vi "sub vi - Read Analog All v9.5.vi"(0 "data 0":waveform(dbl)[](array[waveform]), 5 "data 1":waveform(dbl)[](array[waveform]), 7 "data 2":waveform(dbl)[](array[waveform]), 9 "AI Error":errorcluster[](array[cluster])) -> (2 "Lab05 -1 Offset I":dbl, 3 "array GRAPH":dynamicdata[](array[waveform]), 4 "LAB01":T2, 6 "LAB02":T3, 8 "LAB03":T4, 10 "LAB04":T5, 13 "deg C":dbl, 14 "USB Error":bool[](array[boolean]), 15 "LAB05":T6)   [LabVIEW 2017]
uses:
  program files/Global display 3.vi
  <vilib>/measure/mascope.llb/Amplitude and Levels 1 chan.vi
  <vilib>/measure/NI_MAPro.lvlib
  <vilib>/measure/madcrms.llb/Basic Averaged DC-RMS for N Chan.vi
panel:
  in  "normalized waveform":waveform(dbl)
  in  "Tab Control":T1(tab)
  out "LAB01-2 (PF)":dbl
  out "LAB01-1 (PF)":dbl
  out "LAB01-2 (V)":dbl
  out "LAB01-2 (A)":dbl
  out "LAB01-1 (V)":dbl
  out "LAB01-1 (A)":dbl
  out "LAB01-2 (GRAPH)":dynamicdata(graph)
  out "LAB01-1 (GRAPH)":dynamicdata(graph)
  out "LAB02-2 (PF)":dbl
  out "LAB02-1 (PF)":dbl
  out "LAB02-2 (V)":dbl
  out "LAB02-2 (A)":dbl
  out "LAB02-1 (V)":dbl
  out "LAB02-1 (A)":dbl
  out "LAB02-2 (GRAPH)":dynamicdata(graph)
  out "LAB02-1 (GRAPH)":dynamicdata(graph)
  out "LAB03-2 (PF)":dbl
  out "LAB03-1 (PF)":dbl
  out "LAB03-2 (V)":dbl
  out "LAB03-2 (A)":dbl
  out "LAB03-1 (V)":dbl
  out "LAB03-1 (A)":dbl
  out "LAB03-2 (GRAPH)":dynamicdata(graph)
  out "LAB03-1 (GRAPH)":dynamicdata(graph)
  out "LAB04-2 (PF)":dbl
  out "LAB04-1 (PF)":dbl
  out "LAB04-2 (V)":dbl
  out "LAB04-2 (A)":dbl
  out "LAB04-1 (V)":dbl
  out "LAB04-1 (A)":dbl
  out "LAB04-1 (GRAPH)":dynamicdata(graph)
  out "LAB04-2 (GRAPH)":dynamicdata(graph)
  out "LAB05-2 (PF)":dbl
  out "LAB05-1 (PF)":dbl
  out "LAB05-2 (V)":dbl
  out "LAB05-2 (A)":dbl
  out "LAB05-1 (V)":dbl
  out "LAB05-1 (A)":dbl
  out "LAB05-1 (GRAPH)":dynamicdata(graph)
  out "LAB05-2 (GRAPH)":dynamicdata(graph)
  out "A1 error":errorcluster
  out "array ERROR":errorcluster[](array[cluster])
  out "AI2-OFF":waveform(dbl)[](graph)
  out "AI2-ON":waveform(dbl)[](graph)
  out "AI1-OFF":waveform(dbl)[](graph)
  out "AI1-ON":waveform(dbl)[](graph)
  out "AI0-OFF":waveform(dbl)[](graph)
  out "AI0-ON":waveform(dbl)[](graph)
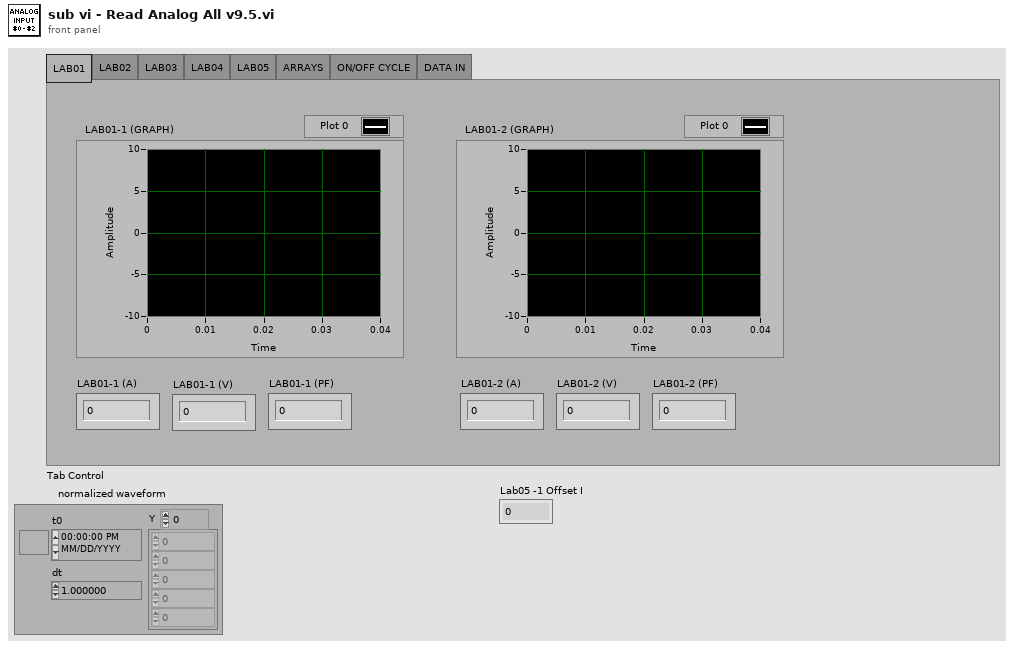
[diagram p1: front panel]
types:
  T1 = enum32{"LAB01", "LAB02", "LAB03", "LAB04", "LAB05", "ARRAYS", "ON/OFF CYCLE", "DATA IN"}
  T2 = cluster{"LAB01-1 (A)":dbl, "LAB01-1 (V)":dbl, "LAB01-1 (PF)":dbl, "LAB01-2 (A)":dbl, "LAB01-2 (V)":dbl, "LAB01-2 (PF)":dbl}
  T3 = cluster{"LAB02-1 (A)":dbl, "LAB02-1 (V)":dbl, "LAB02-1 (PF)":dbl, "LAB02-2 (A)":dbl, "LAB02-2 (V)":dbl, "LAB02-2 (PF)":dbl}
  T4 = cluster{"LAB03-1 (A)":dbl, "LAB03-1 (V)":dbl, "LAB03-1 (PF)":dbl, "LAB03-2 (A)":dbl, "LAB03-2 (V)":dbl, "LAB03-2 (PF)":dbl}
  T5 = cluster{"LAB04-1 (A)":dbl, "LAB04-1 (V)":dbl, "LAB04-1 (PF)":dbl, "LAB04-2 (A)":dbl, "LAB04-2 (V)":dbl, "LAB04-2 (PF)":dbl}
  T6 = cluster{"LAB05-1 (A)":dbl, "LAB05-1 (V)":dbl, "LAB05-1 (PF)":dbl, "LAB05-2 (A)":dbl, "LAB05-2 (V)":dbl, "LAB05-2 (PF)":dbl}
  T7 = cluster{"active power [W]":dbl, "apparent power [VA]":dbl, "reactive power [VAR]":dbl, "power factor":dbl}
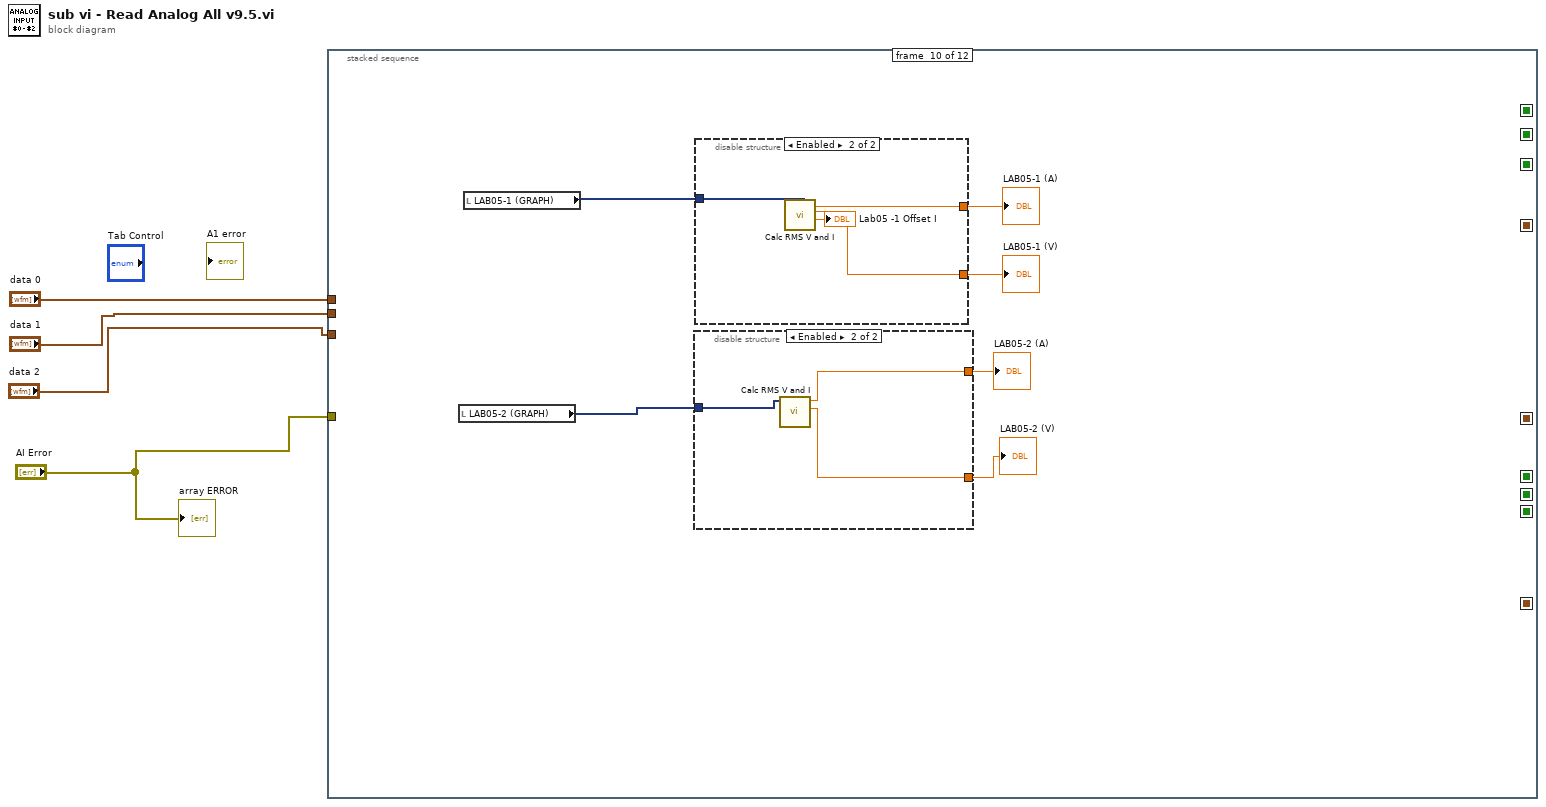
[diagram p0: block diagram]
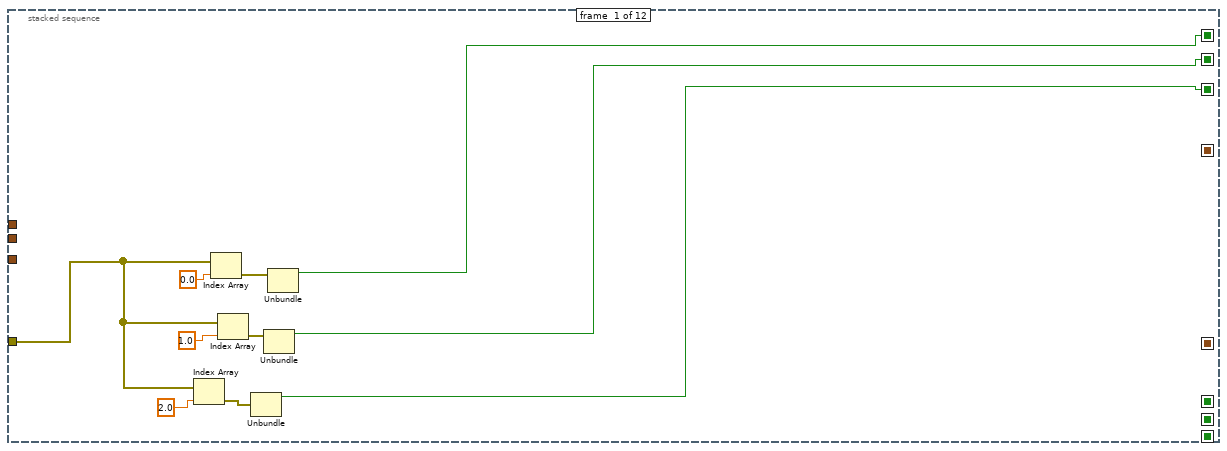
[diagram p2: hidden frame]
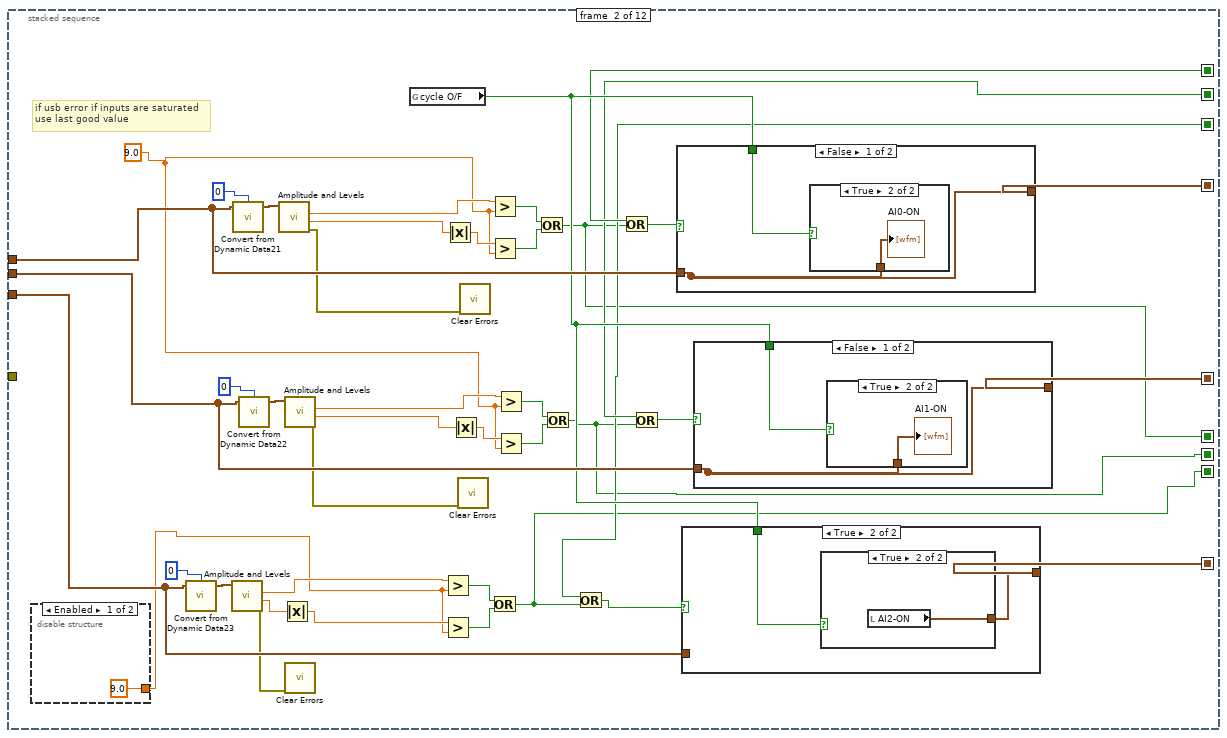
[diagram p3: hidden frame]
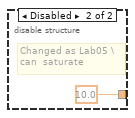
[diagram p4: hidden frame]
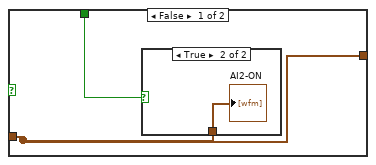
[diagram p5: hidden frame]
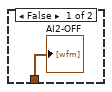
[diagram p6: hidden frame]
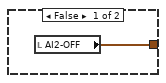
[diagram p7: hidden frame]
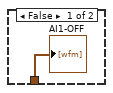
[diagram p8: hidden frame]
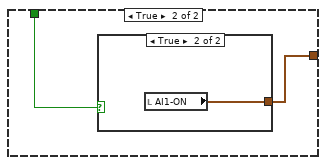
[diagram p9: hidden frame]
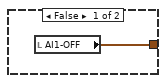
[diagram p10: hidden frame]
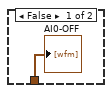
[diagram p11: hidden frame]
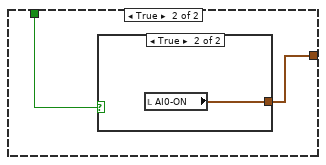
[diagram p12: hidden frame]
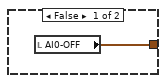
[diagram p13: hidden frame]
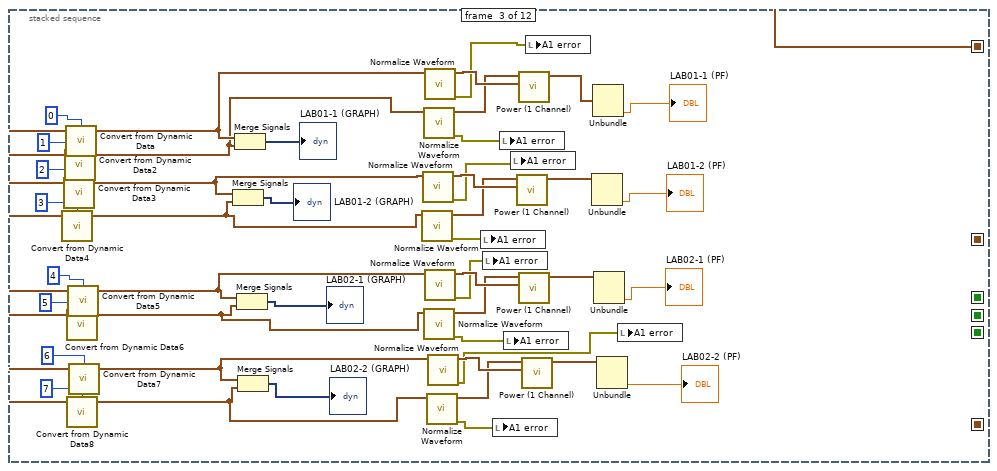
[diagram p14: hidden frame]
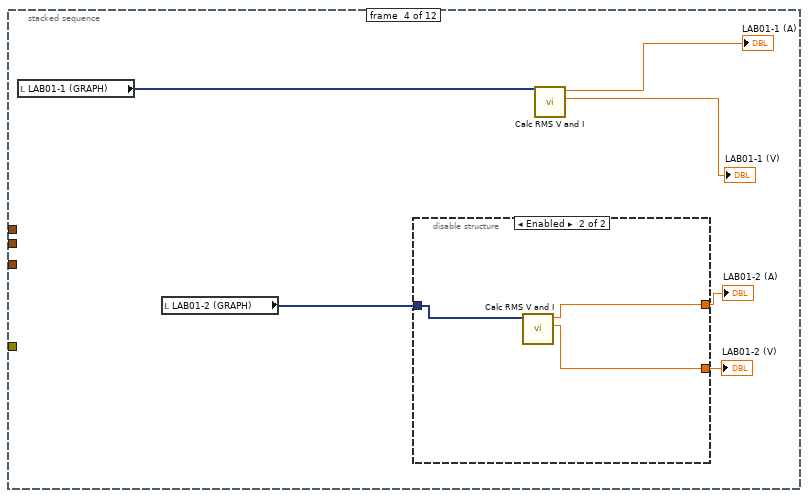
[diagram p15: hidden frame]
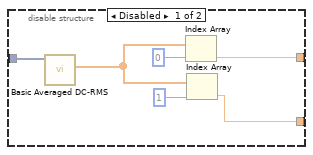
[diagram p16: hidden frame]
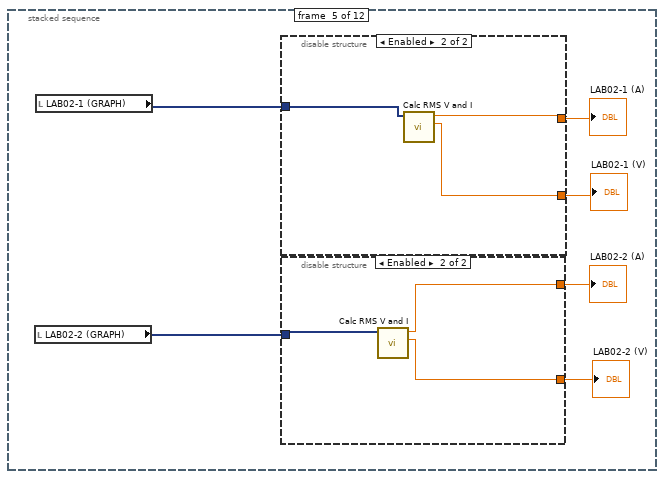
[diagram p17: hidden frame]
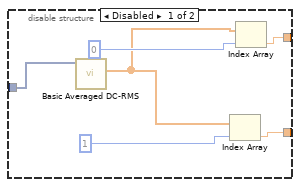
[diagram p18: hidden frame]
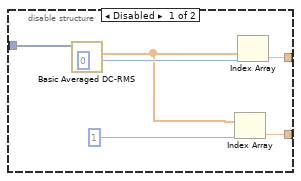
[diagram p19: hidden frame]
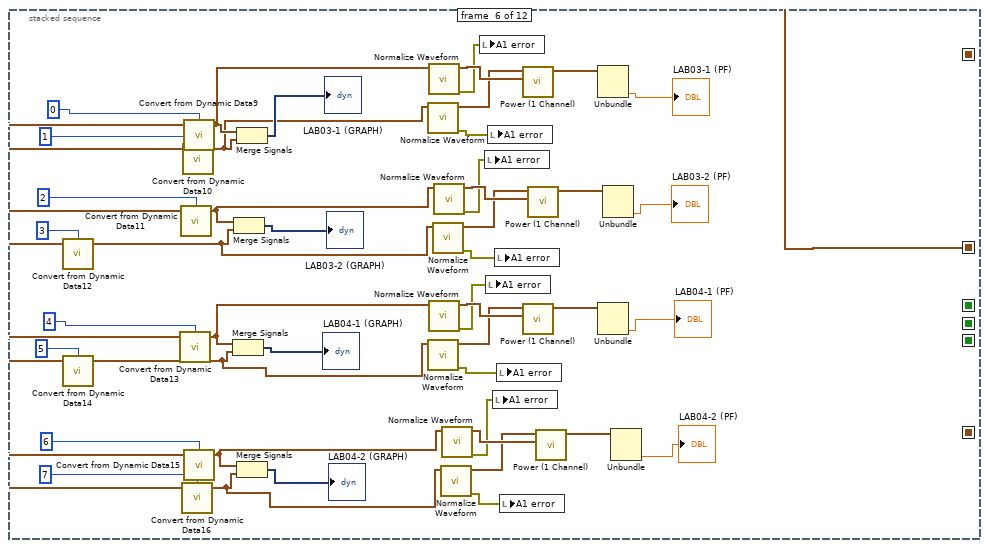
[diagram p20: hidden frame]
diagram:
  n1 = stacked-sequence {
    seq-local: [w12 _ _ _ _ _ _ _ _ _ _ _] -> [_ w24 _ _ _ _ _ _ _ _ _ w327]
    seq-local: [w9 _ _ _ _ _ _ _ _ _ _ _] -> [_ w23 _ _ _ _ _ _ _ _ _ w326]
    seq-local: [w5 _ _ _ _ _ _ _ _ _ _ _] -> [_ w20 _ _ _ _ _ _ _ _ _ w325]
    seq-local: [_ w49 _ _ _ _ _ _ _ _ _ _] -> [_ _ w127 _ _ _ _ _ _ _ _ _]
    seq-local: [_ w39 _ _ _ _ _ _ _ _ _ _] -> [_ _ _ _ _ w211 _ _ _ _ _ _]
    seq-local: [_ w29 _ _ _ _ _ _ _ _ _ _] -> [_ _ _ _ _ _ _ _ w262 _ _ _]
    seq-local: [_ w19 _ _ _ _ _ _ _ _ _ _] -> [_ _ _ _ _ _ _ _ _ _ _ w324]
    seq-local: [_ w18 _ _ _ _ _ _ _ _ _ _] -> [_ _ _ _ _ _ _ _ _ _ _ w323]
    seq-local: [_ w17 _ _ _ _ _ _ _ _ _ _] -> [_ _ _ _ _ _ _ _ _ _ _ w322]
    tunnel: "data 0" -> [_ w48 _ _ _ _ _ _ _ _ _ _]
    tunnel: "data 1" -> [_ w40 _ _ _ _ _ _ _ _ _ _]
    tunnel: "data 2" -> [_ w31 _ _ _ _ _ _ _ _ _ _]
    tunnel: "AI Error" -> [w6 _ _ _ _ _ _ _ _ _ _ _]
    frame #0 {
      n2 = Index Array(array=w6, index=2.0) -> (element=w7:errorcluster)
      n3 = Index Array(array=w6, index=0.0) -> (element=w13:errorcluster)
      n4 = Index Array(array=w6, index=1.0) -> (element=w10:errorcluster)
      n5 = Unbundle(w7) -> ("status"=w5:bool)  [unwired: 2 out]
      n6 = Unbundle(w10) -> ("status"=w9:bool)  [unwired: 2 out]
      n7 = Unbundle(w13) -> ("status"=w12:bool)  [unwired: 2 out]
    }
    frame #1 {
      w15 = 9.0
      # "if usb error if inputs are saturated\nuse last good value"
      n8 = disable-structure shown="Enabled" {
        disable-tunnel: [9.0 10.0] -> w16
        frame Enabled {
        }
        frame Disabled {
          # "Changed as Lab05 \\\ncan  saturate"
        }
      }
      n9 = call "Convert from Dynamic Data23"("Dynamic Data Type"=w31, "Channel"=0) -> ("Waveform"=w37:waveform(dbl))  [unwired: 2 in]
      n10 = call-poly <vilib>:"Amplitude and Levels.vi"("signal in"=w37) -> ("error out"=w26:errorcluster, "low state level"=w36:dbl, "high state level"=w35:dbl)  [unwired: 7 in, 1 out]
      n11 = call "Convert from Dynamic Data21"("Dynamic Data Type"=w48, "Channel"=0) -> ("Waveform"=w55:waveform(dbl))  [unwired: 2 in]
      n12 = call "Convert from Dynamic Data22"("Dynamic Data Type"=w40, "Channel"=0) -> ("Waveform"=w46:waveform(dbl))  [unwired: 2 in]
      n13 = call-poly <vilib>:"Amplitude and Levels.vi"("signal in"=w55) -> ("error out"=w28:errorcluster, "low state level"=w54:dbl, "high state level"=w53:dbl)  [unwired: 7 in, 1 out]
      n14 = Absolute Value(x=w36) -> (abs(x)=w34:dbl)
      n15 = call-poly <vilib>:"Amplitude and Levels.vi"("signal in"=w46) -> ("error out"=w27:errorcluster, "low state level"=w45:dbl, "high state level"=w44:dbl)  [unwired: 7 in, 1 out]
      n16 = call <vilib>:"Clear Errors.vi"("error in (no error)"=w26) -> ()  [unwired: 5 in, 2 out]
      n17 = global read "Global display 3.vi" "cycle O/F"() -> (w30:bool)
      n18 = Greater?(x=w35, y=w16) -> (0:w33:bool)
      n19 = Greater?(x=w34, y=w16) -> (0:w32:bool)
      n20 = Absolute Value(x=w54) -> (abs(x)=w52:dbl)
      n21 = Absolute Value(x=w45) -> (abs(x)=w43:dbl)
      n22 = call <vilib>:"Clear Errors.vi"("error in (no error)"=w27) -> ()  [unwired: 5 in, 2 out]
      n23 = call <vilib>:"Clear Errors.vi"("error in (no error)"=w28) -> ()  [unwired: 5 in, 2 out]
      n24 = Greater?(x=w53, y=w15) -> (0:w51:bool)
      n25 = Greater?(x=w52, y=w15) -> (0:w50:bool)
      n26 = Or(x=w33, y=w32) -> (x .or. y?=w17:bool)
      n27 = Greater?(x=w44, y=w15) -> (0:w42:bool)
      n28 = Greater?(x=w43, y=w15) -> (0:w41:bool)
      n29 = Or(x=w51, y=w50) -> (x .or. y?=w19:bool)
      n30 = Or(x=w42, y=w41) -> (x .or. y?=w18:bool)
      n31 = Or(x=w20, y=w17) -> (x .or. y?=w21:bool)
      n32 = Or(x=w24, y=w19) -> (x .or. y?=w25:bool)
      n33 = Or(x=w23, y=w18) -> (x .or. y?=w22:bool)
      n34 = case shown="False" w25 {
        tunnel: w30 -> [w76 w80]
        tunnel: [w75 w79] -> w49
        tunnel: w48 -> [w75 _]
        frame False {
          n35 = case shown="True" w76 {
            tunnel: w75 -> [w77 w78]
            frame False {
              "AI0-OFF" <- w77
            }
            frame True {
              "AI0-ON" <- w78
            }
          }
        }
        frame True {
          n36 = case shown="True" w80 {
            tunnel: [w81 w82] -> w79
            frame False {
              n37 = local read "AI0-OFF"() -> (w81:waveform(dbl)[])
            }
            frame True {
              n38 = local read "AI0-ON"() -> (w82:waveform(dbl)[])
            }
          }
        }
      }
      n39 = case shown="True" w21 {
        tunnel: w30 -> [w60 w64]
        tunnel: [w59 w63] -> w29
        tunnel: w31 -> [w59 _]
        frame False {
          n40 = case shown="True" w60 {
            tunnel: w59 -> [w61 w62]
            frame False {
              "AI2-OFF" <- w61
            }
            frame True {
              "AI2-ON" <- w62
            }
          }
        }
        frame True {
          n41 = case shown="True" w64 {
            tunnel: [w65 w66] -> w63
            frame False {
              n42 = local read "AI2-OFF"() -> (w65:waveform(dbl)[])
            }
            frame True {
              n43 = local read "AI2-ON"() -> (w66:waveform(dbl)[])
            }
          }
        }
      }
      n44 = case shown="False" w22 {
        tunnel: w30 -> [w68 w72]
        tunnel: [w67 w71] -> w39
        tunnel: w40 -> [w67 _]
        frame False {
          n45 = case shown="True" w68 {
            tunnel: w67 -> [w69 w70]
            frame False {
              "AI1-OFF" <- w69
            }
            frame True {
              "AI1-ON" <- w70
            }
          }
        }
        frame True {
          n46 = case shown="True" w72 {
            tunnel: [w73 w74] -> w71
            frame False {
              n47 = local read "AI1-OFF"() -> (w73:waveform(dbl)[])
            }
            frame True {
              n48 = local read "AI1-ON"() -> (w74:waveform(dbl)[])
            }
          }
        }
      }
    }
    frame #2 {
      n49 = call "Convert from Dynamic Data4"("Dynamic Data Type"=w127, "Channel"=3) -> ("Waveform"=w103:waveform(dbl))  [unwired: 2 in]
      n50 = call "Convert from Dynamic Data3"("Dynamic Data Type"=w127, "Channel"=2) -> ("Waveform"=w104:waveform(dbl))  [unwired: 2 in]
      n51 = call "Convert from Dynamic Data2"("Dynamic Data Type"=w127, "Channel"=1) -> ("Waveform"=w113:waveform(dbl))  [unwired: 2 in]
      n52 = call "Convert from Dynamic Data"("Dynamic Data Type"=w127, "Channel"=0) -> ("Waveform"=w114:waveform(dbl))  [unwired: 2 in]
      n53 = call "Convert from Dynamic Data6"("Dynamic Data Type"=w127, "Channel"=5) -> ("Waveform"=w98:waveform(dbl))  [unwired: 2 in]
      n54 = call "Convert from Dynamic Data8"("Dynamic Data Type"=w127, "Channel"=7) -> ("Waveform"=w92:waveform(dbl))  [unwired: 2 in]
      n55 = call "Convert from Dynamic Data5"("Dynamic Data Type"=w127, "Channel"=4) -> ("Waveform"=w99:waveform(dbl))  [unwired: 2 in]
      n56 = call "Convert from Dynamic Data7"("Dynamic Data Type"=w127, "Channel"=6) -> ("Waveform"=w93:waveform(dbl))  [unwired: 2 in]
      n57 = Merge Signals(w104, w103) -> (→"LAB01-2 (GRAPH)":dynamicdata)
      n58 = Merge Signals(w114, w113) -> (→"LAB01-1 (GRAPH)":dynamicdata)
      n59 = Merge Signals(w99, w98) -> (→"LAB02-1 (GRAPH)":dynamicdata)
      n60 = Merge Signals(w93, w92) -> (→"LAB02-2 (GRAPH)":dynamicdata)
      n61 = call <vilib>:"Normalize Waveform.vi"("waveform in"=w103) -> ("error out"=w87:errorcluster, "normalized waveform"=w107:waveform(dbl))  [unwired: 7 in, 2 out]
      n62 = call <vilib>:"Normalize Waveform.vi"("waveform in"=w104) -> ("error out"=w88:errorcluster, "normalized waveform"=w108:waveform(dbl))  [unwired: 7 in, 2 out]
      n63 = call <vilib>:"Normalize Waveform.vi"("waveform in"=w113) -> ("error out"=w89:errorcluster, "normalized waveform"=w111:waveform(dbl))  [unwired: 7 in, 2 out]
      n64 = call <vilib>:"Normalize Waveform.vi"("waveform in"=w98) -> ("error out"=w85:errorcluster, "normalized waveform"=w101:waveform(dbl))  [unwired: 7 in, 2 out]
      n65 = call <vilib>:"Normalize Waveform.vi"("waveform in"=w114) -> ("error out"=w90:errorcluster, "normalized waveform"=w112:waveform(dbl))  [unwired: 7 in, 2 out]
      n66 = call <vilib>:"Normalize Waveform.vi"("waveform in"=w99) -> ("error out"=w86:errorcluster, "normalized waveform"=w102:waveform(dbl))  [unwired: 7 in, 2 out]
      n67 = call <vilib>:"Normalize Waveform.vi"("waveform in"=w92) -> ("error out"=w83:errorcluster, "normalized waveform"=w95:waveform(dbl))  [unwired: 7 in, 2 out]
      n68 = call <vilib>:"Normalize Waveform.vi"("waveform in"=w93) -> ("error out"=w84:errorcluster, "normalized waveform"=w96:waveform(dbl))  [unwired: 7 in, 2 out]
      n69 = local write "A1 error"(w87) -> ()
      n70 = local write "A1 error"(w86) -> ()
      n71 = local write "A1 error"(w83) -> ()
      n72 = local write "A1 error"(w89) -> ()
      n73 = local write "A1 error"(w85) -> ()
      n74 = local write "A1 error"(w88) -> ()
      n75 = call "Power (1 Channel).vi"("current waveform"=w108, "voltage waveform"=w107) -> ("power value"=w106:T7)  [unwired: 9 in]
      n76 = call "Power (1 Channel).vi"("current waveform"=w112, "voltage waveform"=w111) -> ("power value"=w110:T7)  [unwired: 9 in]
      n77 = call "Power (1 Channel).vi"("current waveform"=w102, "voltage waveform"=w101) -> ("power value"=w100:T7)  [unwired: 9 in]
      n78 = call "Power (1 Channel).vi"("current waveform"=w96, "voltage waveform"=w95) -> ("power value"=w94:T7)  [unwired: 9 in]
      n79 = local write "A1 error"(w90) -> ()
      n80 = Unbundle(w106) -> ("power factor"=→"LAB01-2 (PF)":dbl)  [unwired: 3 out]
      n81 = Unbundle(w110) -> ("power factor"=→"LAB01-1 (PF)":dbl)  [unwired: 3 out]
      n82 = Unbundle(w100) -> ("power factor"=→"LAB02-1 (PF)":dbl)  [unwired: 3 out]
      n83 = Unbundle(w94) -> ("power factor"=→"LAB02-2 (PF)":dbl)  [unwired: 3 out]
      n84 = local write "A1 error"(w84) -> ()
    }
    frame #3 {
      n85 = local read "LAB01-1 (GRAPH)"() -> (w128:dynamicdata)
      n86 = local read "LAB01-2 (GRAPH)"() -> (w129:dynamicdata)
      n87 = disable-structure shown="Enabled" {
        disable-tunnel: [w136 w141] -> w133
        disable-tunnel: [w135 w140] -> w132
        disable-tunnel: w129 -> [w134 w142]
        frame Disabled {
          n88 = call-poly <vilib>:"Basic Averaged DC-RMS.vi"("signals in"=w134) -> ("RMS values"=w139:dbl[])  [unwired: 7 in, 3 out]
          n89 = Index Array(array=w139, index=0) -> (element=w136:dbl)
          n90 = Index Array(array=w139, index=1) -> (element=w135:dbl)
        }
        frame Enabled {
          n91 = call "Calc RMS V and I.vi"("LAB01-1 (GRAPH)"=w142) -> ("RMS V"=w140:dbl, "RMS I"=w141:dbl)  [unwired: 8 in, 1 out]
        }
      }
      "LAB01-2 (A)" <- w133
      "LAB01-2 (V)" <- w132
      n92 = call "Calc RMS V and I.vi"("LAB01-1 (GRAPH)"=w128) -> ("RMS V"=→"LAB01-1 (V)":dbl, "RMS I"=→"LAB01-1 (A)":dbl)  [unwired: 8 in, 1 out]
    }
    frame #4 {
      n93 = local read "LAB02-2 (GRAPH)"() -> (w144:dynamicdata)
      n94 = local read "LAB02-1 (GRAPH)"() -> (w143:dynamicdata)
      n95 = disable-structure shown="Enabled" {
        disable-tunnel: [w160 w165] -> w148
        disable-tunnel: [w159 w164] -> w147
        disable-tunnel: w143 -> [w158 w166]
        frame Disabled {
          n96 = call-poly <vilib>:"Basic Averaged DC-RMS.vi"("signals in"=w158) -> ("RMS values"=w161:dbl[])  [unwired: 7 in, 3 out]
          n97 = Index Array(array=w161, index=1) -> (element=w159:dbl)
          n98 = Index Array(array=w161, index=0) -> (element=w160:dbl)
        }
        frame Enabled {
          n99 = call "Calc RMS V and I.vi"("LAB01-1 (GRAPH)"=w166) -> ("RMS V"=w164:dbl, "RMS I"=w165:dbl)  [unwired: 8 in, 1 out]
        }
      }
      "LAB02-1 (A)" <- w148
      "LAB02-1 (V)" <- w147
      n100 = disable-structure shown="Enabled" {
        disable-tunnel: [w151 w156] -> w146
        disable-tunnel: [w150 w155] -> w145
        disable-tunnel: w144 -> [w149 w157]
        frame Disabled {
          n101 = call-poly <vilib>:"Basic Averaged DC-RMS.vi"("signals in"=w149) -> ("RMS values"=w152:dbl[])  [unwired: 7 in, 3 out]
          n102 = Index Array(array=w152, index=1) -> (element=w150:dbl)
          n103 = Index Array(array=w152, index=0) -> (element=w151:dbl)
        }
        frame Enabled {
          n104 = call "Calc RMS V and I.vi"("LAB01-1 (GRAPH)"=w157) -> ("RMS V"=w155:dbl, "RMS I"=w156:dbl)  [unwired: 8 in, 1 out]
        }
      }
      "LAB02-2 (A)" <- w146
      "LAB02-2 (V)" <- w145
    }
    frame #5 {
      n105 = call "Convert from Dynamic Data12"("Dynamic Data Type"=w211, "Channel"=3) -> ("Waveform"=w188:waveform(dbl))  [unwired: 2 in]
      n106 = call "Convert from Dynamic Data14"("Dynamic Data Type"=w211, "Channel"=5) -> ("Waveform"=w182:waveform(dbl))  [unwired: 2 in]
      n107 = call "Convert from Dynamic Data13"("Dynamic Data Type"=w211, "Channel"=4) -> ("Waveform"=w183:waveform(dbl))  [unwired: 2 in]
      n108 = call "Convert from Dynamic Data11"("Dynamic Data Type"=w211, "Channel"=2) -> ("Waveform"=w189:waveform(dbl))  [unwired: 2 in]
      n109 = call "Convert from Dynamic Data16"("Dynamic Data Type"=w211, "Channel"=7) -> ("Waveform"=w176:waveform(dbl))  [unwired: 2 in]
      n110 = call "Convert from Dynamic Data10"("Dynamic Data Type"=w211, "Channel"=1) -> ("Waveform"=w194:waveform(dbl))  [unwired: 2 in]
      n111 = call "Convert from Dynamic Data9"("Dynamic Data Type"=w211, "Channel"=0) -> ("Waveform"=w195:waveform(dbl))  [unwired: 2 in]
      n112 = call "Convert from Dynamic Data15"("Dynamic Data Type"=w211, "Channel"=6) -> ("Waveform"=w177:waveform(dbl))  [unwired: 2 in]
      n113 = Merge Signals(w183, w182) -> (→"LAB04-1 (GRAPH)":dynamicdata)
      n114 = Merge Signals(w189, w188) -> (→"LAB03-2 (GRAPH)":dynamicdata)
      n115 = Merge Signals(w195, w194) -> (→"LAB03-1 (GRAPH)":dynamicdata)
      n116 = Merge Signals(w177, w176) -> (→"LAB04-2 (GRAPH)":dynamicdata)
      n117 = call <vilib>:"Normalize Waveform.vi"("waveform in"=w194) -> ("error out"=w173:errorcluster, "normalized waveform"=w197:waveform(dbl))  [unwired: 7 in, 2 out]
      n118 = call <vilib>:"Normalize Waveform.vi"("waveform in"=w182) -> ("error out"=w169:errorcluster, "normalized waveform"=w185:waveform(dbl))  [unwired: 7 in, 2 out]
      n119 = call <vilib>:"Normalize Waveform.vi"("waveform in"=w195) -> ("error out"=w174:errorcluster, "normalized waveform"=w198:waveform(dbl))  [unwired: 7 in, 2 out]
      n120 = call <vilib>:"Normalize Waveform.vi"("waveform in"=w183) -> ("error out"=w170:errorcluster, "normalized waveform"=w186:waveform(dbl))  [unwired: 7 in, 2 out]
      n121 = call <vilib>:"Normalize Waveform.vi"("waveform in"=w188) -> ("error out"=w171:errorcluster, "normalized waveform"=w191:waveform(dbl))  [unwired: 7 in, 2 out]
      n122 = call <vilib>:"Normalize Waveform.vi"("waveform in"=w189) -> ("error out"=w172:errorcluster, "normalized waveform"=w192:waveform(dbl))  [unwired: 7 in, 2 out]
      n123 = call <vilib>:"Normalize Waveform.vi"("waveform in"=w176) -> ("error out"=w167:errorcluster, "normalized waveform"=w179:waveform(dbl))  [unwired: 7 in, 2 out]
      n124 = call <vilib>:"Normalize Waveform.vi"("waveform in"=w177) -> ("error out"=w168:errorcluster, "normalized waveform"=w180:waveform(dbl))  [unwired: 7 in, 2 out]
      n125 = local write "A1 error"(w174) -> ()
      n126 = local write "A1 error"(w172) -> ()
      n127 = local write "A1 error"(w170) -> ()
      n128 = local write "A1 error"(w173) -> ()
      n129 = local write "A1 error"(w168) -> ()
      n130 = local write "A1 error"(w171) -> ()
      n131 = local write "A1 error"(w169) -> ()
      n132 = local write "A1 error"(w167) -> ()
      n133 = call "Power (1 Channel).vi"("current waveform"=w198, "voltage waveform"=w197) -> ("power value"=w196:T7)  [unwired: 9 in]
      n134 = call "Power (1 Channel).vi"("current waveform"=w186, "voltage waveform"=w185) -> ("power value"=w184:T7)  [unwired: 9 in]
      n135 = call "Power (1 Channel).vi"("current waveform"=w192, "voltage waveform"=w191) -> ("power value"=w190:T7)  [unwired: 9 in]
      n136 = call "Power (1 Channel).vi"("current waveform"=w180, "voltage waveform"=w179) -> ("power value"=w178:T7)  [unwired: 9 in]
      n137 = Unbundle(w196) -> ("power factor"=→"LAB03-1 (PF)":dbl)  [unwired: 3 out]
      n138 = Unbundle(w184) -> ("power factor"=→"LAB04-1 (PF)":dbl)  [unwired: 3 out]
      n139 = Unbundle(w190) -> ("power factor"=→"LAB03-2 (PF)":dbl)  [unwired: 3 out]
      n140 = Unbundle(w178) -> ("power factor"=→"LAB04-2 (PF)":dbl)  [unwired: 3 out]
    }
    frame #6 {
      n141 = local read "LAB03-2 (GRAPH)"() -> (w212:dynamicdata)
      n142 = local read "LAB03-1 (GRAPH)"() -> (w213:dynamicdata)
      n143 = disable-structure shown="Enabled" {
        disable-tunnel: [w220 w224] -> w215
        disable-tunnel: [w219 w225] -> w214
        disable-tunnel: w212 -> [w218 w226]
        frame Disabled {
          n144 = call-poly <vilib>:"Basic Averaged DC-RMS.vi"("signals in"=w218) -> ("RMS values"=w221:dbl[])  [unwired: 7 in, 3 out]
          n145 = Index Array(array=w221, index=0) -> (element=w219:dbl)
          n146 = Index Array(array=w221, index=1) -> (element=w220:dbl)
        }
        frame Enabled {
          n147 = call "Calc RMS V and I.vi"("LAB01-1 (GRAPH)"=w226) -> ("RMS V"=w224:dbl, "RMS I"=w225:dbl)  [unwired: 8 in, 1 out]
        }
      }
      "LAB03-2 (A)" <- w214
      "LAB03-2 (V)" <- w215
      n148 = disable-structure shown="Enabled" {
        disable-tunnel: [w229 w234] -> w217
        disable-tunnel: [w228 w233] -> w216
        disable-tunnel: w213 -> [w227 w235]
        frame Disabled {
          n149 = call-poly <vilib>:"Basic Averaged DC-RMS.vi"("signals in"=w227) -> ("RMS values"=w230:dbl[])  [unwired: 7 in, 3 out]
          n150 = Index Array(array=w230, index=0) -> (element=w229:dbl)
          n151 = Index Array(array=w230, index=1) -> (element=w228:dbl)
        }
        frame Enabled {
          n152 = call "Calc RMS V and I.vi"("LAB01-1 (GRAPH)"=w235) -> ("RMS V"=w233:dbl, "RMS I"=w234:dbl)  [unwired: 8 in, 1 out]
        }
      }
      "LAB03-1 (A)" <- w217
      "LAB03-1 (V)" <- w216
    }
    frame #7 {
      n153 = local read "LAB04-2 (GRAPH)"() -> (w236:dynamicdata)
      n154 = local read "LAB04-1 (GRAPH)"() -> (w237:dynamicdata)
      n155 = disable-structure shown="Enabled" {
        disable-tunnel: [w244 w248] -> w239
        disable-tunnel: [w243 w249] -> w238
        disable-tunnel: w236 -> [w242 w250]
        frame Disabled {
          n156 = call-poly <vilib>:"Basic Averaged DC-RMS.vi"("signals in"=w242) -> ("RMS values"=w245:dbl[])  [unwired: 7 in, 3 out]
          n157 = Index Array(array=w245, index=0) -> (element=w243:dbl)
          n158 = Index Array(array=w245, index=1) -> (element=w244:dbl)
        }
        frame Enabled {
          n159 = call "Calc RMS V and I.vi"("LAB01-1 (GRAPH)"=w250) -> ("RMS V"=w248:dbl, "RMS I"=w249:dbl)  [unwired: 8 in, 1 out]
        }
      }
      "LAB04-2 (A)" <- w238
      "LAB04-2 (V)" <- w239
      n160 = disable-structure shown="Enabled" {
        disable-tunnel: [w253 w258] -> w241
        disable-tunnel: [w252 w257] -> w240
        disable-tunnel: w237 -> [w251 w259]
        frame Disabled {
          n161 = call-poly <vilib>:"Basic Averaged DC-RMS.vi"("signals in"=w251) -> ("RMS values"=w254:dbl[])  [unwired: 7 in, 3 out]
          n162 = Index Array(array=w254, index=0) -> (element=w253:dbl)
          n163 = Index Array(array=w254, index=1) -> (element=w252:dbl)
        }
        frame Enabled {
          n164 = call "Calc RMS V and I.vi"("LAB01-1 (GRAPH)"=w259) -> ("RMS V"=w257:dbl, "RMS I"=w258:dbl)  [unwired: 8 in, 1 out]
        }
      }
      "LAB04-1 (A)" <- w241
      "LAB04-1 (V)" <- w240
    }
    frame #8 {
      n165 = call "Convert from Dynamic Data18"("Dynamic Data Type"=w262, "Channel"=1) -> ("Waveform"=w276:waveform(dbl))  [unwired: 2 in]
      n166 = call "Convert from Dynamic Data20"("Dynamic Data Type"=w262, "Channel"=3) -> ("Waveform"=w270:waveform(dbl))  [unwired: 2 in]
      n167 = call "Convert from Dynamic Data17"("Dynamic Data Type"=w262, "Channel"=0) -> ("Waveform"=w277:waveform(dbl))  [unwired: 2 in]
      n168 = call "Convert from Dynamic Data19"("Dynamic Data Type"=w262, "Channel"=2) -> ("Waveform"=w271:waveform(dbl))  [unwired: 2 in]
      n169 = Merge Signals(w277, w276) -> (→"LAB05-1 (GRAPH)":dynamicdata)
      n170 = Merge Signals(w271, w270) -> (→"LAB05-2 (GRAPH)":dynamicdata)
      n171 = call "Convert from Dynamic Data24"("Dynamic Data Type"=w262, "Channel"=4) -> ("Waveform"=w261:waveform(dbl))  [unwired: 2 in]
      n172 = call "RMS.vi"("current waveform"=w261) -> ("RMS"=→"deg C":dbl)  [unwired: 10 in]
      n173 = call <vilib>:"Normalize Waveform.vi"("waveform in"=w276) -> ("error out"=w268:errorcluster, "normalized waveform"=w278:waveform(dbl))  [unwired: 7 in, 2 out]
      n174 = call <vilib>:"Normalize Waveform.vi"("waveform in"=w277) -> ("error out"=w267:errorcluster, "normalized waveform"=w279:waveform(dbl))  [unwired: 7 in, 2 out]
      n175 = call <vilib>:"Normalize Waveform.vi"("waveform in"=w270) -> ("error out"=w266:errorcluster, "normalized waveform"=w273:waveform(dbl))  [unwired: 7 in, 2 out]
      n176 = call <vilib>:"Normalize Waveform.vi"("waveform in"=w271) -> ("error out"=w265:errorcluster, "normalized waveform"=w274:waveform(dbl))  [unwired: 7 in, 2 out]
      n177 = local write "A1 error"(w266) -> ()
      n178 = local write "A1 error"(w267) -> ()
      n179 = local write "A1 error"(w265) -> ()
      n180 = call "Power (1 Channel).vi"("current waveform"=w279, "voltage waveform"=w278) -> ("power value"=w263:T7)  [unwired: 9 in]
      n181 = local write "A1 error"(w268) -> ()
      n182 = call "Power (1 Channel).vi"("current waveform"=w274, "voltage waveform"=w273) -> ("power value"=w272:T7)  [unwired: 9 in]
      n183 = Unbundle By Name(w263) -> ("power factor"=→"LAB05-1 (PF)":dbl)  [unwired: 3 out]
      n184 = Unbundle(w272) -> ("power factor"=→"LAB05-2 (PF)":dbl)  [unwired: 3 out]
    }
    frame #9 {
      n185 = local read "LAB05-2 (GRAPH)"() -> (w286:dynamicdata)
      n186 = local read "LAB05-1 (GRAPH)"() -> (w287:dynamicdata)
      n187 = disable-structure shown="Enabled" {
        disable-tunnel: [w294 w299] -> w291
        disable-tunnel: [w293 w298] -> w290
        disable-tunnel: w286 -> [w292 w300]
        frame Disabled {
          n188 = call-poly <vilib>:"Basic Averaged DC-RMS.vi"("signals in"=w292) -> ("RMS values"=w295:dbl[])  [unwired: 7 in, 3 out]
          n189 = Index Array(array=w295, index=1) -> (element=w293:dbl)
          n190 = Index Array(array=w295, index=0) -> (element=w294:dbl)
        }
        frame Enabled {
          n191 = call "Calc RMS V and I.vi"("LAB01-1 (GRAPH)"=w300) -> ("RMS V"=w298:dbl, "RMS I"=w299:dbl)  [unwired: 8 in, 1 out]
        }
      }
      "LAB05-2 (A)" <- w291
      "LAB05-2 (V)" <- w290
      n192 = disable-structure shown="Enabled" {
        disable-tunnel: [w303 w309] -> w289
        disable-tunnel: [w302 w308] -> w288
        disable-tunnel: w287 -> [w301 w310]
        frame Disabled {
          n193 = call-poly <vilib>:"Basic Averaged DC-RMS.vi"("signals in"=w301) -> ("RMS values"=w304:dbl[])  [unwired: 7 in, 3 out]
          n194 = Index Array(array=w304, index=1) -> (element=w302:dbl)
          n195 = Index Array(array=w304, index=0) -> (element=w303:dbl)
        }
        frame Enabled {
          n196 = call "Calc RMS V and I.vi"("LAB01-1 (GRAPH)"=w310) -> ("Offset I"=→"Lab05 -1 Offset I":dbl, "RMS V"=w308:dbl, "RMS I"=w309:dbl)  [unwired: 8 in]
        }
      }
      "LAB05-1 (A)" <- w289
      "LAB05-1 (V)" <- w288
    }
    frame #10 {
      n197 = local read "LAB05-1 (GRAPH)"() -> (w313:dynamicdata)
      n198 = local read "LAB05-2 (GRAPH)"() -> (w312:dynamicdata)
      n199 = local read "LAB04-2 (GRAPH)"() -> (w314:dynamicdata)
      n200 = local read "LAB02-2 (GRAPH)"() -> (w318:dynamicdata)
      n201 = local read "LAB03-1 (GRAPH)"() -> (w317:dynamicdata)
      n202 = local read "LAB04-1 (GRAPH)"() -> (w315:dynamicdata)
      n203 = local read "LAB03-2 (GRAPH)"() -> (w316:dynamicdata)
      n204 = local read "LAB02-1 (GRAPH)"() -> (w319:dynamicdata)
      n205 = local read "LAB01-2 (GRAPH)"() -> (w320:dynamicdata)
      n206 = local read "LAB01-1 (GRAPH)"() -> (w321:dynamicdata)
      n207 = Build Array(w321, w320, w319, w318, w317, w316, w315, w314, w313, w312) -> (→"array GRAPH":dynamicdata[])
    }
    frame #11 {
      n208 = local read "LAB03-2 (PF)"() -> (w346:dbl)
      n209 = local read "LAB03-1 (PF)"() -> (w349:dbl)
      n210 = local read "LAB03-1 (A)"() -> (w351:dbl)
      n211 = local read "LAB03-1 (V)"() -> (w350:dbl)
      n212 = local read "LAB03-2 (A)"() -> (w348:dbl)
      n213 = local read "LAB03-2 (V)"() -> (w347:dbl)
      n214 = local read "LAB01-1 (PF)"() -> (w356:dbl)
      n215 = local read "LAB01-2 (PF)"() -> (w353:dbl)
      n216 = local read "LAB01-1 (V)"() -> (w357:dbl)
      n217 = local read "LAB01-2 (A)"() -> (w355:dbl)
      n218 = local read "LAB01-2 (V)"() -> (w354:dbl)
      n219 = local read "LAB01-1 (A)"() -> (w358:dbl)
      n220 = Bundle("LAB03-1 (A)"=w351, "LAB03-1 (V)"=w350, "LAB03-1 (PF)"=w349, "LAB03-2 (A)"=w348, "LAB03-2 (V)"=w347, "LAB03-2 (PF)"=w346) -> (→"LAB03":T4)  [unwired: 1 in]
      n221 = local read "LAB05-2 (PF)"() -> (w332:dbl)
      n222 = local read "LAB05-1 (PF)"() -> (w335:dbl)
      n223 = Bundle("LAB01-1 (A)"=w358, "LAB01-1 (V)"=w357, "LAB01-1 (PF)"=w356, "LAB01-2 (A)"=w355, "LAB01-2 (V)"=w354, "LAB01-2 (PF)"=w353) -> (→"LAB01":T2)  [unwired: 1 in]
      n224 = local read "LAB05-2 (V)"() -> (w333:dbl)
      n225 = local read "LAB05-1 (A)"() -> (w337:dbl)
      n226 = local read "LAB05-1 (V)"() -> (w336:dbl)
      n227 = local read "LAB05-2 (A)"() -> (w334:dbl)
      n228 = local read "LAB04-1 (PF)"() -> (w343:dbl)
      n229 = local read "LAB04-2 (PF)"() -> (w340:dbl)
      n230 = local read "LAB04-1 (A)"() -> (w345:dbl)
      n231 = local read "LAB04-1 (V)"() -> (w344:dbl)
      n232 = local read "LAB04-2 (A)"() -> (w342:dbl)
      n233 = local read "LAB04-2 (V)"() -> (w341:dbl)
      n234 = local read "LAB02-2 (PF)"() -> (w360:dbl)
      n235 = local read "LAB02-1 (PF)"() -> (w363:dbl)
      n236 = local read "LAB02-2 (A)"() -> (w362:dbl)
      n237 = local read "LAB02-2 (V)"() -> (w361:dbl)
      n238 = local read "LAB02-1 (V)"() -> (w364:dbl)
      n239 = local read "LAB02-1 (A)"() -> (w365:dbl)
      n240 = Bundle("LAB05-1 (A)"=w337, "LAB05-1 (V)"=w336, "LAB05-1 (PF)"=w335, "LAB05-2 (A)"=w334, "LAB05-2 (V)"=w333, "LAB05-2 (PF)"=w332) -> (→"LAB05":T6)  [unwired: 1 in]
      n241 = Bundle("LAB04-1 (A)"=w345, "LAB04-1 (V)"=w344, "LAB04-1 (PF)"=w343, "LAB04-2 (A)"=w342, "LAB04-2 (V)"=w341, "LAB04-2 (PF)"=w340) -> (→"LAB04":T5)  [unwired: 1 in]
      n242 = Bundle("LAB02-1 (A)"=w365, "LAB02-1 (V)"=w364, "LAB02-1 (PF)"=w363, "LAB02-2 (A)"=w362, "LAB02-2 (V)"=w361, "LAB02-2 (PF)"=w360) -> (→"LAB02":T3)  [unwired: 1 in]
      n243 = Or(x=w326, y=w323) -> (x .or. y?=w328:bool)
      n244 = Or(x=w327, y=w322) -> (x .or. y?=w330:bool)
      n245 = Or(x=w325, y=w324) -> (x .or. y?=w329:bool)
      n246 = Build Array(w330, w328, w329) -> (→"USB Error":bool[])
    }
  }
  "array ERROR" <- "AI Error"
